vi "Reserve Sessions.vi"(6 "timeout (ms)":i32, 8 "error in":errorcluster, 9 "instrument type id":string, 10 "pin or relay names":string[](array[string]), 11 "pin map context":T1) -> (0 "error out":errorcluster, 3 "session reservation out":refnum<class "Session Reservation.lvclass">)   [LabVIEW 2020, in "MeasurementLink Session Management.lvlib" / "Session Reservation.lvclass"]
doc: "Reserves session(s) based on the provided instrument type and pin information."
uses:
  Session Reservation.lvclass
  MeasurementLink Session Management Client/RPC Messages/ni_measurementlink_PinMapContext.ctl
  MeasurementLink Session Management Client/MeasurementLink Session Management Client.lvlib
  MeasurementLink Session Management Client/RPC Messages/ni_measurementlink_sessionmanagement_v1_ReserveSessionsRequest.ctl
  MeasurementLink gRPC Utilities/gRPC Client Pool/gRPC Client Pool.lvclass
  MeasurementLink gRPC Utilities/gRPC Client Pool/FGV Action.ctl
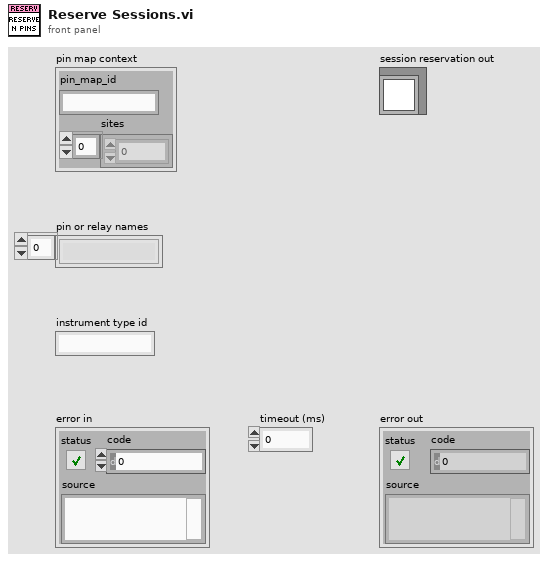
[diagram p1: front panel]
types:
  T1 = typedef "MeasurementLink Session Management Client.lvlib/ni_measurementlink_PinMapContext.ctl" = cluster{"pin_map_id":string, "sites":i32[]}
  T2 = typedef "MeasurementLink gRPC Utilities.lvlib/gRPC Client Pool.lvclass/FGV Action.ctl" = enum16{"Get Discovery Client", "Get Session Client", "Get Pinmap Client", "Destroy Clients"}
  T3 = typedef "MeasurementLink Session Management Client.lvlib/ni_measurementlink_sessionmanagement_v1_ReserveSessionsRequest.ctl" = cluster{"pin_map_context":T1, "pin_or_relay_names":string[], "instrument_type_id":string, "timeout_in_milliseconds":i32}
  T4 = typedef "grpc-lvsupport-release.lvlib/grpcId.ctl" = u64
  T5 = typedef "MeasurementLink Session Management Client.lvlib/ni_measurementlink_sessionmanagement_v1_ReserveSessionsResponse.ctl" = cluster{"sessions":T6[]}
  T6 = typedef "MeasurementLink Session Management Client.lvlib/ni_measurementlink_sessionmanagement_v1_SessionInformation.ctl" = cluster{"session":T7, "resource_name":string, "channel_list":string, "instrument_type_id":string, "session_exists":bool, "channel_mappings":T8[]}
  T7 = typedef "MeasurementLink Session Management Client.lvlib/nidevice_grpc_Session.ctl" = cluster{"name":string}
  T8 = typedef "MeasurementLink Session Management Client.lvlib/ni_measurementlink_sessionmanagement_v1_ChannelMapping.ctl" = cluster{"pin_or_relay_name":string, "site":i32, "channel":string}
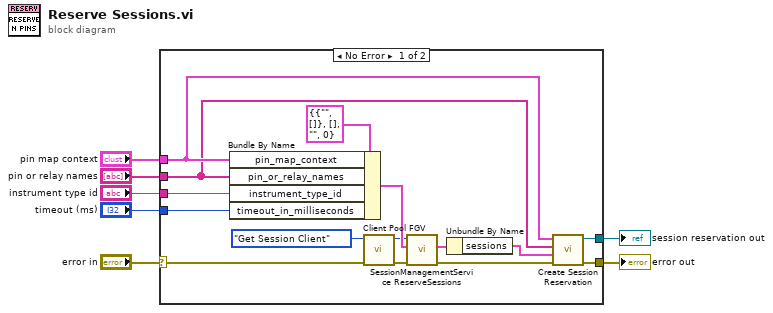
[diagram p0: block diagram]
diagram:
  n1 = case shown="No Error" "error in" {
    selector: "error in" -> [w17 w23]
    tunnel: "instrument type id" -> [w16 _]
    tunnel: "pin or relay names" -> [w9 _]
    tunnel: "timeout (ms)" -> [w15 _]
    tunnel: "pin map context" -> [w10 _]
    tunnel: [w12 w23] -> w3
    tunnel: [w11 _] -> w1
    frame No Error {
      n2 = Bundle By Name(cluster=T3 {"pin_map_context"={"pin_map_id"="", "sites"=[]}, "pin_or_relay_names"=[], "instrument_type_id"="", "timeout_in_milliseconds"=0} ("Request Data"), "pin_map_context"=w10, "pin_or_relay_names"=w9, "instrument_type_id"=w16, "timeout_in_milliseconds"=w15) -> (w21:T3)
      n3 = call "Client Pool FGV.vi"("error in (no error)"=w17, "Action"=FGV_Action."Get Session Client") -> ("error out"=w19:errorcluster, "grpc client id"=w18:T4)  [unwired: 8 in]
      n4 = call "SessionManagementService ReserveSessions.vi"("error in"=w19, "Request Data"=w21, "gRPC ID"=w18) -> ("error out"=w13:errorcluster, "Response Data"=w14:T5)  [unwired: 6 in, 1 out]
      n5 = Unbundle By Name(w14) -> ("sessions"=w8:T6[])
      n6 = call "Create Session Reservation.vi"("pin map context"=w10, "pin or relay names"=w9, "sessions"=w8, "error in (no error)"=w13) -> ("session reservation out"=w11:refnum<class "Session Reservation.lvclass">, "error out"=w12:errorcluster)  [unwired: 5 in]
    }
    frame Error {
    }
  }
  "session reservation out" <- w1
  "error out" <- w3
